vi "serial_09.vi"(0 "VISA resource name":refnum<visa-resource-name>="COM4") -> ()   [LabVIEW 2010]
doc: "The Basic Serial Read and Write example performs a Serial Port Read, a Serial Port Write, or a combination of these actions. The user selects the actions (read or write) on the front panel. If both are selected, the VI will write the data first, read data, and then close the VISA session that is opened to the port. This VI will wait until the specified number of bytes is received at the port. Only the number of bytes specified will be read.\n\nINSTRUCTIONS:\n1) Select the serial resource and configuration parameters (baud rate, data bits, parity, stop bits, flow control).\n2) Select the operations to be performed. \n3) Connect the serial port to your device. If no device is available, perform a loopback test by doing one of the following. Short pins 2 and 3 on a RS-232 cable or short pin 4 to pin 8 and pin 5 to pin 9 on a RS-485/422 cable. \n4) Run the VI to see the data read. (The \"read string\" will match the \"string to write\" if a loopback test was performed.)\n\nNote: The parameters set for the serial port must match the parameters of the connected instrument or device. In this example, the bytes to read parameter specifies the number of bytes that the serial port reads. If there were more bytes at the port than the number specified in bytes to read, those bytes would not be read. Also, if you specify to read more bytes than the number of bytes actually read, you might receive a timeout error message.\n\nOn the block diagram, the Configure Serial Port VI sets the configuration parameters. The front panel displays the controls used to configure the basic parameters, such as baud rate, data bits, and parity. Constants configure the other parameters the user probably does not need set. After the VISA Configure Serial Port VI opens the VISA session and configures the port, the VI passes the VISA resource name to other VIs that perform operations on that VISA resource. The VISA Write function sends a command to the serial device and the VISA Read function returns data based on the command. The VISA Close function then closes the reference to the serial device. It is important to close the reference; otherwise communication through with that port through protocols other than VISA might not be possible."
panel:
  out "Comanda":string="O1"
  in  "Leduri":bool[](array[boolean])=[FALSE, FALSE, FALSE, FALSE, FALSE, FALSE, FALSE, TRUE]
  in  "Start":bool=TRUE
  # "Stop"
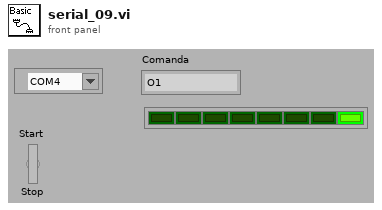
[diagram p1: front panel]
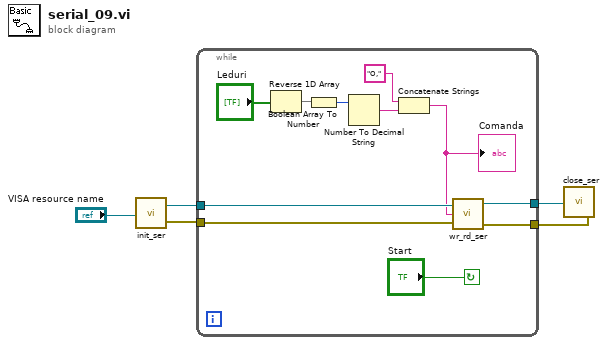
[diagram p0: block diagram]
diagram:
  n1 = call "init_ser.vi"("VISA resource name"="VISA resource name") -> ("VISA resource name out"=w3:refnum<visa-resource-name>, "error out"=w4:errorcluster)
  n2 = while {
    tunnel: w4 -> [w14]
    tunnel: w3 -> [w15]
    tunnel: [w12] -> w2
    tunnel: [w13] -> w1
    stop <- "Start" continue-if-true
    n3 = Reverse 1D Array(array="Leduri") -> (reversed array=w7:bool[])
    n4 = Boolean Array To Number(Boolean array=w7) -> (number=w6:u32)
    n5 = Number To Decimal String(number=w6) -> (decimal integer string=w10:string)  [unwired: 1 in]
    n6 = Concatenate Strings("O,", w10) -> (w11:string)
    "Comanda" <- w11
    n7 = call "wr_rd_ser.vi"("error in"=w14, "string to write"=w11, "VISA resource name in"=w15) -> ("error out"=w12:errorcluster, "VISA resource name out"=w13:refnum<visa-resource-name>)  [unwired: 1 out]
  }
  n8 = call "close_ser.vi"("error in"=w2, "VISA resource name in"=w1) -> ()
